vi "Set Next Actor.vi"(8 "error in (no error)":errorcluster, 10 "Message Enqueuer":refnum<class "Message Enqueuer.lvclass">, 11 "Pipelined Actor in":refnum<class "Pipelined Actor.lvclass">) -> (0 "error out":errorcluster, 3 "Pipelined Actor out":refnum<class "Pipelined Actor.lvclass">)   [LabVIEW 2014, in "Pipelined Actor.lvlib" / "Pipelined Actor.lvclass"]
uses:
  Pipelined Actor.lvclass
  <vilib>/ActorFramework/Message Enqueuer/Message Enqueuer.lvclass
  Pipelined Actor.lvclass/Pipelined Actor.ctl
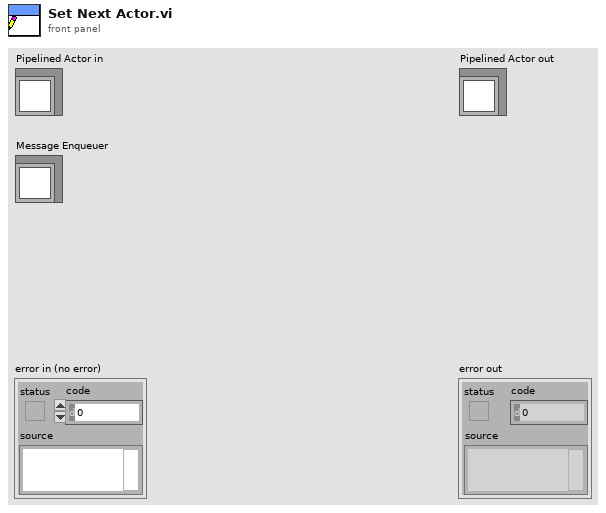
[diagram p1: front panel]
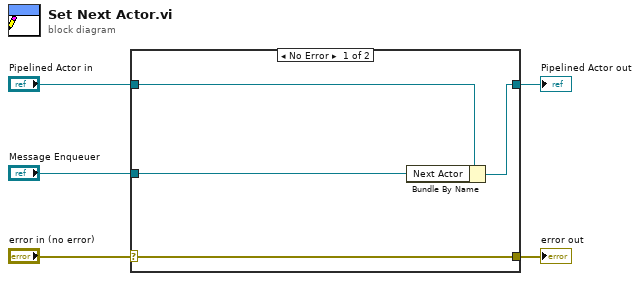
[diagram p0: block diagram]
diagram:
  n1 = case shown="No Error" "error in (no error)" {
    selector: "error in (no error)" -> [w9 w10]
    tunnel: [w9 w10] -> w4
    tunnel: [w7 w11] -> w2
    tunnel: "Pipelined Actor in" -> [w8 w11]
    tunnel: "Message Enqueuer" -> [w6 _]
    frame No Error {
      n2 = Bundle By Name(cluster=w8, "Next Actor"=w6) -> (w7:refnum<class "Pipelined Actor.lvclass">)
    }
    frame Error {
    }
  }
  "error out" <- w4
  "Pipelined Actor out" <- w2
